vi "CAN_update.vi"(10 "布尔":bool, 11 "VI输入":refnum<vi>) -> ()   [LabVIEW 2018, in "UI.lvlib"]
uses:
  controls/UI.lvlib
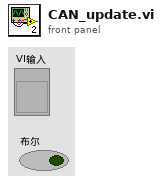
[diagram p1: front panel]
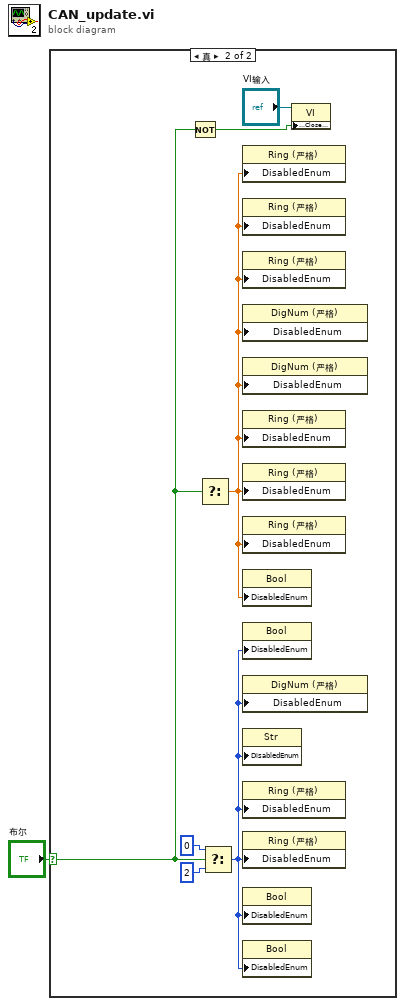
[diagram p0: block diagram]
diagram:
  n1 = case shown="真" "布尔" {
    selector: "布尔" -> [_ w2]
    frame False {
    }
    frame True {
      n2 = Not(x=w2) -> (.not. x?=w6:bool)
      n3 = Select(s=w2) -> (s? t:f=w8:dbl)  [unwired: 2 in]
      n4 = Select(t=0, s=w2, f=2) -> (s? t:f=w7:i32)
      n5 = property on="属性节点" class="Ring (严格)"("DisabledEnum"=w8) -> ()  [unwired: 2 in, 2 out]
      n6 = property on="属性节点" class="Ring (严格)"("DisabledEnum"=w8) -> ()  [unwired: 2 in, 2 out]
      n7 = property on="属性节点" class="Ring (严格)"("DisabledEnum"=w8) -> ()  [unwired: 2 in, 2 out]
      n8 = property on="属性节点" class="DigNum (严格)"("DisabledEnum"=w8) -> ()  [unwired: 2 in, 2 out]
      n9 = property on="属性节点" class="DigNum (严格)"("DisabledEnum"=w8) -> ()  [unwired: 2 in, 2 out]
      n10 = property on="属性节点" class="Ring (严格)"("DisabledEnum"=w8) -> ()  [unwired: 2 in, 2 out]
      n11 = property on="属性节点" class="Ring (严格)"("DisabledEnum"=w8) -> ()  [unwired: 2 in, 2 out]
      n12 = property on="属性节点" class="Ring (严格)"("DisabledEnum"=w8) -> ()  [unwired: 2 in, 2 out]
      n13 = property on="属性节点" class="Bool"("DisabledEnum"=w8) -> ()  [unwired: 2 in, 2 out]
      n14 = property on="属性节点" class="Bool"("DisabledEnum"=w7) -> ()  [unwired: 2 in, 2 out]
      n15 = property on="属性节点" class="DigNum (严格)"("DisabledEnum"=w7) -> ()  [unwired: 2 in, 2 out]
      n16 = property on="属性节点" class="Str"("DisabledEnum"=w7) -> ()  [unwired: 2 in, 2 out]
      n17 = property on="属性节点" class="Ring (严格)"("DisabledEnum"=w7) -> ()  [unwired: 2 in, 2 out]
      n18 = property on="属性节点" class="Ring (严格)"("DisabledEnum"=w7) -> ()  [unwired: 2 in, 2 out]
      n19 = property on="属性节点" class="Bool"("DisabledEnum"=w7) -> ()  [unwired: 2 in, 2 out]
      n20 = property on="属性节点" class="Bool"("DisabledEnum"=w7) -> ()  [unwired: 2 in, 2 out]
      n21 = property class="VI"(reference="VI输入", "Front Panel.Closeable"=w6) -> ()  [unwired: 1 in, 2 out]
    }
  }
